vi "BRig_Host__Loop_Producer__tcp_System__Data_saveClosedLoopCmdList.vi"(10 "input_I_SentCmd":bool, 11 "input_filepath_storage":string) -> ()   [LabVIEW 2014]
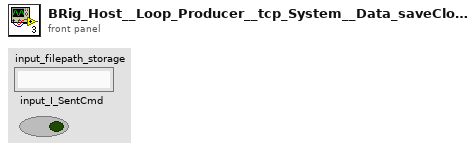
[diagram p1: front panel]
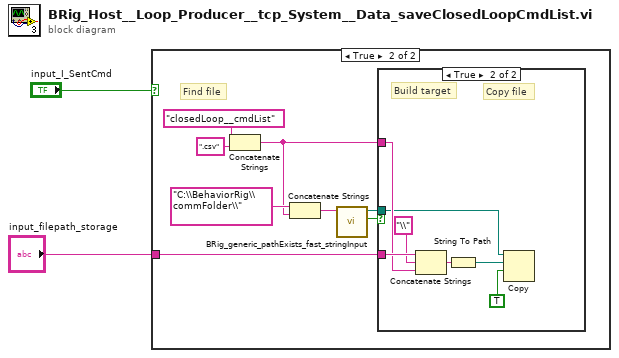
[diagram p0: block diagram]
diagram:
  n1 = case shown="True" "input_I_SentCmd" {
    tunnel: "input_filepath_storage" -> [_ w5]
    frame False {
    }
    frame True {
      # "Find file"
      n2 = Concatenate Strings("closedLoop__cmdList" ("string"), ".csv" ("string")) -> (w4:string)
      n3 = Concatenate Strings("C:\\BehaviorRig\\commFolder\\", w4) -> (w7:string)
      n4 = call "BRig_generic_pathExists_fast_stringInput.vi"("input_filePath"=w7) -> ("output_Iexist"=w6:bool, "output_filePath"=w3:path)  [unwired: 8 in, 1 out]
      n5 = case shown="True" w6 {
        tunnel: w5 -> [_ w17]
        tunnel: w4 -> [_ w16]
        tunnel: w3 -> [_ w14]
        frame False {
        }
        frame True {
          # "Copy file"
          # "Build target"
          n6 = Concatenate Strings(w17, "\\" ("string"), w16) -> (w13:string)
          n7 = String To Path(string=w13) -> (path=w12:path)
          n8 = Copy(9:TRUE ("overwrite (F)"), 10:w12, 11:w14) -> ()  [unwired: 2 in, 3 out]
        }
      }
    }
  }
